vi "Pulse Attribute, Get Numeric Results.vi"(4 "error in":errorcluster, 6 "results":T1[](array[typedef])=[{"Label"="Stim Amp (mA)", "Value"=nan}, {"Label"="Stim Pulse Width (us)", "Value"=nan}, {"Label"="Interphase Delay (us)", "Value"=nan}, {"Label"="Recvy Amp (mA)", "Value"=nan}, {"Label"="Recvy Pulse Width (us)", "Value"=nan}, {"Label"="Frequency (Hz)", "Value"=nan}, {"Label"="Period Jitter (us rms)", "Value"=nan}] {"Value" format="%#.3f"}) -> (0 "error out":errorcluster, 2 "numeric values":dbl[](array[numeric]))   [LabVIEW 2010]
doc: "This function extracts Pulse Attribute test results from an array of clusters to an array of doubles."
uses:
  Generic/Waveform Attribute/Waveform Attribute Cluster.ctl
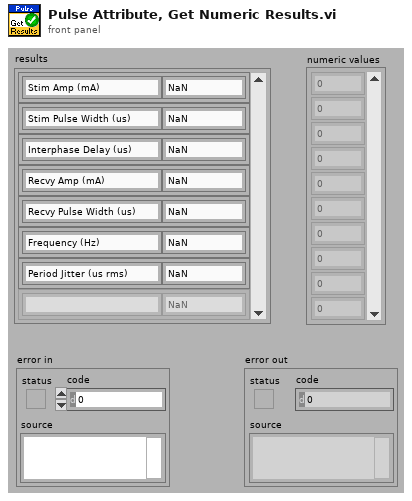
[diagram p1: front panel]
types:
  T1 = typedef "Waveform Attribute Cluster.ctl" = cluster{"Label":string, "Value":dbl}
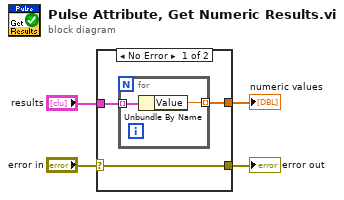
[diagram p0: block diagram]
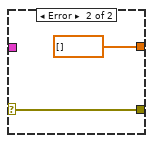
[diagram p2: hidden frame]
diagram:
  n1 = case shown="No Error" "error in" {
    selector: "error in" -> [w5 w11]
    tunnel: [w5 w11] -> w3
    tunnel: "results" -> [w7 _]
    tunnel: [w6 dbl[] []] -> w1
    frame No Error {
      n2 = for {
        tunnel: w7 -> [w9] mode=indexing
        tunnel: [w8] -> w6 mode=indexing
        n3 = Unbundle By Name(w9) -> ("Value"=w8:dbl)
      }
    }
    frame Error {
    }
  }
  "error out" <- w3
  "numeric values" <- w1
